vi "logDpData.vi"(0 "psiplot":cluster{"Double":dbl, "y_r":dbl, "y":dbl}, 4 "yplot":cluster{"Double":dbl, "y_r":dbl, "y":dbl}, 6 "xplot":cluster{"Double":dbl, "y_r":dbl, "y":dbl}, 8 "e_i":dbl[](array[numeric]), 9 "e_b":dbl[](array[numeric]), 10 "time":dbl, 11 "dpPath":path) -> ()   [LabVIEW 2014]
uses:
  <vilib>/Utility/file.llb/Write To Spreadsheet File (DBL).vi
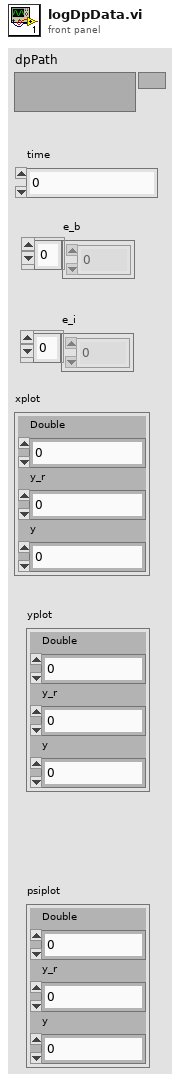
[diagram p1: front panel]
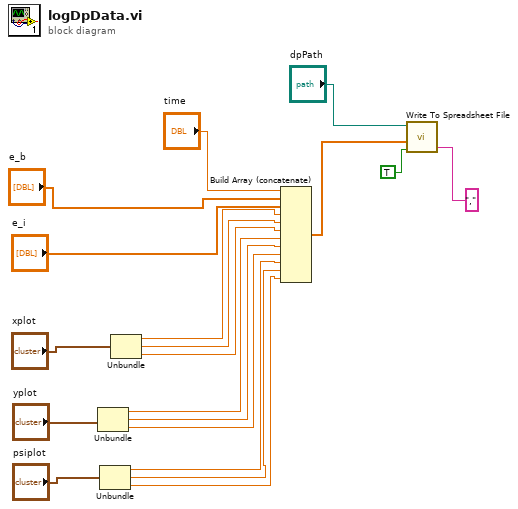
[diagram p0: block diagram]
diagram:
  n1 = Unbundle("yplot") -> ("Double"=w6:dbl, "y_r"=w5:dbl, "y"=w4:dbl)
  n2 = Unbundle("psiplot") -> ("Double"=w3:dbl, "y_r"=w2:dbl, "y"=w1:dbl)
  n3 = Unbundle("xplot") -> ("Double"=w9:dbl, "y_r"=w8:dbl, "y"=w7:dbl)
  n4 = Build Array (concatenate)("time", "e_b", "e_i", w9, w8, w7, w6, w5, w4, w3, w2, w1) -> (w18:dbl[])
  n5 = call-poly <vilib>:"Write To Spreadsheet File.vi"("delimiter (\\t)"="," ("delimiter (\\t)"), "append to file? (new file:F)"=TRUE, "1D data"=w18, "file path (dialog if empty)"="dpPath") -> ()  [unwired: 4 in, 1 out]
